vi "FindTDMSLogs.vi"(8 "error in (no error)":errorcluster, 11 "Directory to search":path) -> (0 "error out":errorcluster, 2 "TDMS Files":path[](array[path]), 3 "Directory to search out":path)   [LabVIEW 2010, in "TDMS to ASCII Convert.lvlib"]
uses:
  TDMS to ASCII Convert.lvlib
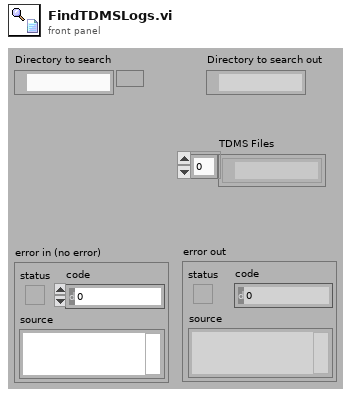
[diagram p1: front panel]
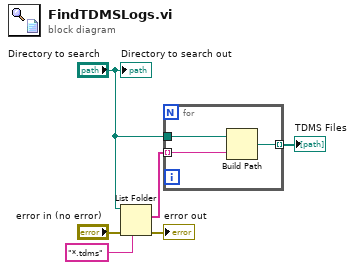
[diagram p0: block diagram]
diagram:
  n1 = List Folder(path="Directory to search", pattern="*.tdms", error in="error in (no error)") -> (filenames=w4:string[], error out=→"error out":errorcluster)  [unwired: 1 in, 2 out]
  n2 = for {
    tunnel: w4 -> [w8] mode=indexing
    tunnel: "Directory to search" -> [w9]
    tunnel: [w7] -> w2 mode=indexing
    n3 = Build Path(base path=w9, name or relative path=w8) -> (appended path=w7:path)
  }
  "TDMS Files" <- w2
  "Directory to search out" <- "Directory to search"
